vi "Auton Position Enum.vi"(8 "Position":T1(ring)) -> (0 "Position":T1(ring))   [LabVIEW 2015]
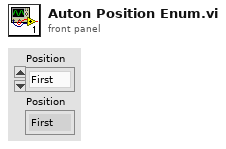
[diagram p1: front panel]
types:
  T1 = enum16{"First", "Second", "Third", "Fourth", "Fifth"}
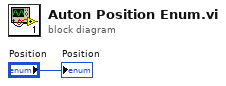
[diagram p0: block diagram]
diagram:
  "Position" <- "Position"
